vi "GeoData.vi"() -> ()   [LabVIEW 2017] (continued)
VA\tAppomattox County\tH1\n22205\t51013\tArlington\tVA\tArlington County\tH1\n22230\t51013\tArlington\tVA\tArlington County\tH1\n22203\t51013\tArlington\tVA\tArlington County\tH1\n22211\t51013\tFort myer\tVA\tArlington County\tH1\n20350\t51013\tWashington\tVA\tArlington County\tH1\n22217\t51013\tArlington\tVA\tArlington County\tH1\n20310\t51013\tWashington\tVA\tArlington County\tH1\n22225\t51013\tArlington\tVA\tArlington County\tH1\n22212\t51013\tArlington\tVA\tArlington County\tH1\n22101\t51013\tMc lean\tVA\tArlington County\tH1\n22202\t51013\tArlington\tVA\tArlington County\tH1\n22204\t51013\tArlington\tVA\tArlington County\tH1\n22243\t51013\tArlington\tVA\tArlington County\tH1\n22046\t51013\tFalls church\tVA\tArlington County\tH1\n22201\t51013\tArlington\tVA\tArlington County\tH1\n22240\t51013\tArlington\tVA\tArlington County\tH1\n20598\t51013\tDhs\tVA\tArlington County\tH1\n22213\t51013\tArlington\tVA\tArlington County\tH1\n22219\t51013\tArlington\tVA\tArlington County\tH1\n22214\t51013\tArlington\tVA\tArlington County\tH1\n22226\t51013\tArlington\tVA\tArlington County\tH1\n22206\t51013\tArlington\tVA\tArlington County\tH1\n22207\t51013\tArlington\tVA\tArlington County\tH1\n22216\t51013\tArlington\tVA\tArlington County\tH1\n22210\t51013\tArlington\tVA\tArlington County\tH1\n22242\t51013\tArlington\tVA\tArlington County\tH1\n22244\t51013\tArlington\tVA\tArlington County\tH1\n20406\t51013\tWashington\tVA\tArlington County\tH1\n22209\t51013\tArlington\tVA\tArlington County\tH1\n20330\t51013\tWashington\tVA\tArlington County\tH1\n22215\t51013\tArlington\tVA\tArlington County\tH1\n20301\t51013\tWashington\tVA\tArlington County\tH1\n22227\t51013\tArlington\tVA\tArlington County\tH1\n22245\t51013\tArlington\tVA\tArlington County\tH1\n22241\t51013\tArlington\tVA\tArlington County\tH1\n22920\t51015\tAfton\tVA\tAugusta County\tH1\n22967\t51015\tRoseland\tVA\tAugusta County\tH1\n24477\t51015\tStuarts draft\tVA\tAugusta County\tH1\n24437\t51015\tFort defiance\tVA\tAugusta County\tH1\n22843\t51015\tMount solon\tVA\tAugusta County\tH1\n22841\t51015\tMount crawford\tVA\tAugusta County\tH1\n24467\t51015\tMount sidney\tVA\tAugusta County\tH1\n24486\t51015\tWeyers cave\tVA\tAugusta County\tH1\n24482\t51015\tVerona\tVA\tAugusta County\tH1\n24483\t51015\tVesuvius\tVA\tAugusta County\tH1\n24440\t51015\tGreenville\tVA\tAugusta County\tH1\n24463\t51015\tMint spring\tVA\tAugusta County\tH1\n22812\t51015\tBridgewater\tVA\tAugusta County\tH1\n22980\t51015\tWaynesboro\tVA\tAugusta County\tH1\n24441\t51015\tGrottoes\tVA\tAugusta County\tH1\n24479\t51015\tSwoope\tVA\tAugusta County\tH1\n22952\t51015\tLyndhurst\tVA\tAugusta County\tH1\n24472\t51015\tRaphine\tVA\tAugusta County\tH1\n24411\t51015\tAugusta springs\tVA\tAugusta County\tH1\n24401\t51015\tStaunton\tVA\tAugusta County\tH1\n24459\t51015\tMiddlebrook\tVA\tAugusta County\tH1\n24421\t51015\tChurchville\tVA\tAugusta County\tH1\n22939\t51015\tFishersville\tVA\tAugusta County\tH1\n24485\t51015\tWest augusta\tVA\tAugusta County\tH1\n24430\t51015\tCraigsville\tVA\tAugusta County\tH1\n24476\t51015\tSteeles tavern\tVA\tAugusta County\tH1\n24469\t51015\tNew hope\tVA\tAugusta County\tH1\n24439\t51015\tGoshen\tVA\tAugusta County\tH1\n24432\t51015\tDeerfield\tVA\tAugusta County\tH1\n24431\t51015\tCrimora\tVA\tAugusta County\tH1\n24460\t51017\tMillboro\tVA\tBath County\tH1\n24422\t51017\tClifton forge\tVA\tBath County\tH1\n24445\t51017\tHot springs\tVA\tBath County\tH1\n24412\t51017\tBacova\tVA\tBath County\tH1\n24487\t51017\tWilliamsville\tVA\tBath County\tH1\n24484\t51017\tWarm springs\tVA\tBath County\tH1\n24432\t51017\tDeerfield\tVA\tBath County\tH1\n24104\t51019\tHuddleston\tVA\tBedford County\tH1\n24122\t51019\tMontvale\tVA\tBedford County\tH1\n24139\t51019\tPittsville\tVA\tBedford County\tH1\n24503\t51019\tLynchburg\tVA\tBedford County\tH1\n24536\t51019\tColeman falls\tVA\tBedford County\tH1\n24523\t51019\tBedford\tVA\tBedford County\tH1\n24550\t51019\tEvington\tVA\tBedford County\tH1\n24101\t51019\tHardy\tVA\tBedford County\tH1\n24179\t51019\tVinton\tVA\tBedford County\tH1\n24502\t51019\tLynchburg\tVA\tBedford County\tH1\n24570\t51019\tLowry\tVA\tBedford County\tH1\n24064\t51019\tBlue ridge\tVA\tBedford County\tH1\n24174\t51019\tThaxton\tVA\tBedford County\tH1\n24501\t51019\tLynchburg\tVA\tBedford County\tH1\n24556\t51019\tGoode\tVA\tBedford County\tH1\n24095\t51019\tGoodview\tVA\tBedford County\tH1\n24551\t51019\tForest\tVA\tBedford County\tH1\n24571\t51019\tLynch station\tVA\tBedford County\tH1\n24121\t51019\tMoneta\tVA\tBedford County\tH1\n24526\t51019\tBig island\tVA\tBedford County\tH1\n24084\t51021\tDublin\tVA\tBland County\tH1\n24315\t51021\tBland\tVA\tBland County\tH1\n24314\t51021\tBastian\tVA\tBland County\tH1\n24124\t51021\tNarrows\tVA\tBland County\tH1\n24134\t51021\tPearisburg\tVA\tBland County\tH1\n24366\t51021\tRocky gap\tVA\tBland County\tH1\n24318\t51021\tCeres\tVA\tBland County\tH1\n24012\t51023\tRoanoke\tVA\tBotetourt County\tH1\n24090\t51023\tFincastle\tVA\tBotetourt County\tH1\n24175\t51023\tTroutville\tVA\tBotetourt County\tH1\n24579\t51023\tNatural bridge station\tVA\tBotetourt County\tH1\n24066\t51023\tBuchanan\tVA\tBotetourt County\tH1\n24450\t51023\tLexington\tVA\tBotetourt County\tH1\n24085\t51023\tEagle rock\tVA\tBotetourt County\tH1\n24422\t51023\tClifton forge\tVA\tBotetourt County\tH1\n24077\t51023\tCloverdale\tVA\tBotetourt County\tH1\n24083\t51023\tDaleville\tVA\tBotetourt County\tH1\n24064\t51023\tBlue ridge\tVA\tBotetourt County\tH1\n24019\t51023\tRoanoke\tVA\tBotetourt County\tH1\n24155\t51023\tRoanoke\tVA\tBotetourt County\tH1\n24130\t51023\tOriskany\tVA\tBotetourt County\tH1\n24438\t51023\tGlen wilton\tVA\tBotetourt County\tH1\n23887\t51025\tValentines\tVA\tBrunswick County\tH1\n23843\t51025\tDolphin\tVA\tBrunswick County\tH1\n23845\t51025\tEbony\tVA\tBrunswick County\tH1\n23873\t51025\tMeredithville\tVA\tBrunswick County\tH1\n23919\t51025\tBracey\tVA\tBrunswick County\tH1\n23856\t51025\tFreeman\tVA\tBrunswick County\tH1\n23847\t51025\tEmporia\tVA\tBrunswick County\tH1\n23876\t51025\tRawlings\tVA\tBrunswick County\tH1\n23868\t51025\tLawrenceville\tVA\tBrunswick County\tH1\n23889\t51025\tWarfield\tVA\tBrunswick County\tH1\n23893\t51025\tWhite plains\tVA\tBrunswick County\tH1\n23920\t51025\tBrodnax\tVA\tBrunswick County\tH1\n23938\t51025\tDundas\tVA\tBrunswick County\tH1\n23824\t51025\tBlackstone\tVA\tBrunswick County\tH1\n23950\t51025\tLa crosse\tVA\tBrunswick County\tH1\n23857\t51025\tGasburg\tVA\tBrunswick County\tH1\n23821\t51025\tAlberta\tVA\tBrunswick County\tH1\n24634\t51027\tPilgrims knob\tVA\tBuchanan County\tH1\n24631\t51027\tOakwood\tVA\tBuchanan County\tH1\n24603\t51027\tBig rock\tVA\tBuchanan County\tH1\n24256\t51027\tHaysi\tVA\tBuchanan County\tH1\n24620\t51027\tHurley\tVA\tBuchanan County\tH1\n24622\t51027\tJewell ridge\tVA\tBuchanan County\tH1\n24656\t51027\tVansant\tVA\tBuchanan County\tH1\n24657\t51027\tWhitewood\tVA\tBuchanan County\tH1\n24639\t51027\tRaven\tVA\tBuchanan County\tH1\n24628\t51027\tMaxie\tVA\tBuchanan County\tH1\n24658\t51027\tWolford\tVA\tBuchanan County\tH1\n24614\t51027\tGrundy\tVA\tBuchanan County\tH1\n24260\t51027\tHonaker\tVA\tBuchanan County\tH1\n24217\t51027\tBee\tVA\tBuchanan County\tH1\n24649\t51027\tSwords creek\tVA\tBuchanan County\tH1\n24646\t51027\tRowe\tVA\tBuchanan County\tH1\n24239\t51027\tDavenport\tVA\tBuchanan County\tH1\n24624\t51027\tKeen mountain\tVA\tBuchanan County\tH1\n24627\t51027\tMavisdale\tVA\tBuchanan County\tH1\n23936\t51029\tDillwyn\tVA\tBuckingham County\tH1\n23921\t51029\tBuckingham\tVA\tBuckingham County\tH1\n24599\t51029\tWingina\tVA\tBuckingham County\tH1\n23901\t51029\tFarmville\tVA\tBuckingham County\tH1\n23004\t51029\tArvonia\tVA\tBuckingham County\tH1\n23123\t51029\tNew canton\tVA\tBuckingham County\tH1\n23040\t51029\tCumberland\tVA\tBuckingham County\tH1\n24522\t51029\tAppomattox\tVA\tBuckingham County\tH1\n24562\t51029\tHowardsville\tVA\tBuckingham County\tH1\n24553\t51029\tGladstone\tVA\tBuckingham County\tH1\n24590\t51029\tScottsville\tVA\tBuckingham County\tH1\n24504\t51031\tLynchburg\tVA\tCampbell County\tH1\n24588\t51031\tRustburg\tVA\tCampbell County\tH1\n24593\t51031\tSpout spring\tVA\tCampbell County\tH1\n24550\t51031\tEvington\tVA\tCampbell County\tH1\n24502\t51031\tLynchburg\tVA\tCampbell County\tH1\n24538\t51031\tConcord\tVA\tCampbell County\tH1\n24554\t51031\tGladys\tVA\tCampbell County\tH1\n24522\t51031\tAppomattox\tVA\tCampbell County\tH1\n24501\t51031\tLynchburg\tVA\tCampbell County\tH1\n24528\t51031\tBrookneal\tVA\tCampbell County\tH1\n24517\t51031\tAltavista\tVA\tCampbell County\tH1\n24576\t51031\tNaruna\tVA\tCampbell County\tH1\n24551\t51031\tForest\tVA\tCampbell County\tH1\n24569\t51031\tLong island\tVA\tCampbell County\tH1\n24571\t51031\tLynch station\tVA\tCampbell County\tH1\n23963\t51031\tRed house\tVA\tCampbell County\tH1\n22427\t51033\tBowling green\tVA\tCaroline County\tH1\n22438\t51033\tChamplain\tVA\tCaroline County\tH1\n22408\t51033\tFredericksburg\tVA\tCaroline County\tH1\n22514\t51033\tMilford\tVA\tCaroline County\tH1\n22560\t51033\tTappahannock\tVA\tCaroline County\tH1\n22436\t51033\tCaret\tVA\tCaroline County\tH1\n22535\t51033\tPort royal\tVA\tCaroline County\tH1\n22552\t51033\tSparta\tVA\tCaroline County\tH1\n22546\t51033\tRuther glen\tVA\tCaroline County\tH1\n22446\t51033\tCorbin\tVA\tCaroline County\tH1\n22580\t51033\tWoodford\tVA\tCaroline County\tH1\n22501\t51033\tLadysmith\tVA\tCaroline County\tH1\n23015\t51033\tBeaverdam\tVA\tCaroline County\tH1\n23047\t51033\tDoswell\tVA\tCaroline County\tH1\n22428\t51033\tBowling green\tVA\tCaroline County\tH1\n23069\t51033\tHanover\tVA\tCaroline County\tH1\n22538\t51033\tRappahannock academy\tVA\tCaroline County\tH1\n24330\t51035\tFries\tVA\tCarroll County\tH1\n24360\t51035\tMax meadows\tVA\tCarroll County\tH1\n24333\t51035\tGalax\tVA\tCarroll County\tH1\n24317\t51035\tCana\tVA\tCarroll County\tH1\n24328\t51035\tFancy gap\tVA\tCarroll County\tH1\n24352\t51035\tLaurel fork\tVA\tCarroll County\tH1\n24053\t51035\tArarat\tVA\tCarroll County\tH1\n24105\t51035\tIndian valley\tVA\tCarroll County\tH1\n24347\t51035\tHiwassee\tVA\tCarroll County\tH1\n24350\t51035\tIvanhoe\tVA\tCarroll County\tH1\n24343\t51035\tHillsville\tVA\tCarroll County\tH1\n24120\t51035\tMeadows of dan\tVA\tCarroll County\tH1\n24325\t51035\tDugspur\tVA\tCarroll County\tH1\n24312\t51035\tAustinville\tVA\tCarroll County\tH1\n24380\t51035\tWillis\tVA\tCarroll County\tH1\n24381\t51035\tWoodlawn\tVA\tCarroll County\tH1\n24351\t51035\tLambsburg\tVA\tCarroll County\tH1\n23030\t51036\tCharles city\tVA\tCharles City County\tH1\n23185\t51036\tWilliamsburg\tVA\tCharles City County\tH1\n23147\t51036\tRuthville\tVA\tCharles City County\tH1\n23231\t51036\tHenrico\tVA\tCharles City County\tH1\n23140\t51036\tProvidence forge\tVA\tCharles City County\tH1\n23937\t51037\tDrakes branch\tVA\tCharlotte County\tH1\n23959\t51037\tPhenix\tVA\tCharlotte County\tH1\n23967\t51037\tSaxe\tVA\tCharlotte County\tH1\n23962\t51037\tRandolph\tVA\tCharlotte County\tH1\n23947\t51037\tKeysville\tVA\tCharlotte County\tH1\n23934\t51037\tCullen\tVA\tCharlotte County\tH1\n23924\t51037\tChase city\tVA\tCharlotte County\tH1\n24522\t51037\tAppomattox\tVA\tCharlotte County\tH1\n24528\t51037\tBrookneal\tVA\tCharlotte County\tH1\n23964\t51037\tRed oak\tVA\tCharlotte County\tH1\n23927\t51037\tClarksville\tVA\tCharlotte County\tH1\n23976\t51037\tWylliesburg\tVA\tCharlotte County\tH1\n23923\t51037\tCharlotte court house\tVA\tCharlotte County\tH1\n23958\t51037\tPamplin\tVA\tCharlotte County\tH1\n23963\t51037\tRed house\tVA\tCharlotte County\tH1\n23224\t51041\tRichmond\tVA\tChesterfield County\tH1\n23235\t51041\tRichmond\tVA\tChesterfield County\tH1\n23834\t51041\tColonial heights\tVA\tChesterfield County\tH1\n23113\t51041\tMidlothian\tVA\tChesterfield County\tH1\n23114\t51041\tMidlothian\tVA\tChesterfield County\tH1\n23112\t51041\tMidlothian\tVA\tChesterfield County\tH1\n23236\t51041\tRichmond\tVA\tChesterfield County\tH1\n23803\t51041\tPetersburg\tVA\tChesterfield County\tH1\n23838\t51041\tChesterfield\tVA\tChesterfield County\tH1\n23120\t51041\tMoseley\tVA\tChesterfield County\tH1\n23832\t51041\tChesterfield\tVA\tChesterfield County\tH1\n23234\t51041\tRichmond\tVA\tChesterfield County\tH1\n23831\t51041\tChester\tVA\tChesterfield County\tH1\n23836\t51041\tChester\tVA\tChesterfield County\tH1\n23225\t51041\tRichmond\tVA\tChesterfield County\tH1\n23237\t51041\tRichmond\tVA\tChesterfield County\tH1\n23297\t51041\tRichmond\tVA\tChesterfield County\tH1\n22630\t51043\tFront royal\tVA\tClarke County\tH1\n20135\t51043\tBluemont\tVA\tClarke County\tH1\n20130\t51043\tParis\tVA\tClarke County\tH1\n22611\t51043\tBerryville\tVA\tClarke County\tH1\n22620\t51043\tBoyce\tVA\tClarke County\tH1\n22663\t51043\tWhite post\tVA\tClarke County\tH1\n22646\t51043\tMillwood\tVA\tClarke County\tH1\n24128\t51045\tNewport\tVA\tCraig County\tH1\n24127\t51045\tNew castle\tVA\tCraig County\tH1\n24070\t51045\tCatawba\tVA\tCraig County\tH1\n24131\t51045\tPaint bank\tVA\tCraig County\tH1\n24426\t51045\tCovington\tVA\tCraig County\tH1\n20186\t51047\tWarrenton\tVA\tCulpeper County\tH1\n22718\t51047\tElkwood\tVA\tCulpeper County\tH1\n22726\t51047\tLignum\tVA\tCulpeper County\tH1\n22714\t51047\tBrandy station\tVA\tCulpeper County\tH1\n20106\t51047\tAmissville\tVA\tCulpeper County\tH1\n22736\t51047\tRichardsville\tVA\tCulpeper County\tH1\n22733\t51047\tRapidan\tVA\tCulpeper County\tH1\n22729\t51047\tMitchells\tVA\tCulpeper County\tH1\n22716\t51047\tCastleton\tVA\tCulpeper County\tH1\n22724\t51047\tJeffersonton\tVA\tCulpeper County\tH1\n22713\t51047\tBoston\tVA\tCulpeper County\tH1\n22701\t51047\tCulpeper\tVA\tCulpeper County\tH1\n22735\t51047\tReva\tVA\tCulpeper County\tH1\n22734\t51047\tRemington\tVA\tCulpeper County\tH1\n22741\t51047\tStevensburg\tVA\tCulpeper County\tH1\n22740\t51047\tSperryville\tVA\tCulpeper County\tH1\n22407\t51047\tFredericksburg\tVA\tCulpeper County\tH1\n22737\t51047\tRixeyville\tVA\tCulpeper County\tH1\n23936\t51049\tDillwyn\tVA\tCumberland County\tH1\n23027\t51049\tCartersville\tVA\tCumberland County\tH1\n23901\t51049\tFarmville\tVA\tCumberland County\tH1\n23038\t51049\tColumbia\tVA\tCumberland County\tH1\n23123\t51049\tNew canton\tVA\tCumberland County\tH1\n23040\t51049\tCumberland\tVA\tCumberland County\tH1\n23139\t51049\tPowhatan\tVA\tCumberland County\tH1\n24237\t51051\tDante\tVA\tDickenson County\tH1\n24230\t51051\tCoeburn\tVA\tDickenson County\tH1\n24220\t51051\tBirchleaf\tVA\tDickenson County\tH1\n24226\t51051\tClinchco\tVA\tDickenson County\tH1\n24256\t51051\tHaysi\tVA\tDickenson County\tH1\n24225\t51051\tCleveland\tVA\tDickenson County\tH1\n24283\t51051\tSaint paul\tVA\tDickenson County\tH1\n24607\t51051\tBreaks\tVA\tDickenson County\tH1\n24656\t51051\tVansant\tVA\tDickenson County\tH1\n24228\t51051\tClintwood\tVA\tDickenson County\tH1\n24217\t51051\tBee\tVA\tDickenson County\tH1\n24272\t51051\tNora\tVA\tDickenson County\tH1\n24269\t51051\tMc clure\tVA\tDickenson County\tH1\n23833\t51053\tChurch road\tVA\tDinwiddie County\tH1\n23803\t51053\tPetersburg\tVA\tDinwiddie County\tH1\n23840\t51053\tDewitt\tVA\tDinwiddie County\tH1\n23805\t51053\tPetersburg\tVA\tDinwiddie County\tH1\n23885\t51053\tSutherland\tVA\tDinwiddie County\tH1\n23872\t51053\tMc kenney\tVA\tDinwiddie County\tH1\n23824\t51053\tBlackstone\tVA\tDinwiddie County\tH1\n23882\t51053\tStony creek\tVA\tDinwiddie County\tH1\n23894\t51053\tWilsons\tVA\tDinwiddie County\tH1\n23850\t51053\tFord\tVA\tDinwiddie County\tH1\n23830\t51053\tCarson\tVA\tDinwiddie County\tH1\n23841\t51053\tDinwiddie\tVA\tDinwiddie County\tH1\n22438\t51057\tChamplain\tVA\tEssex County\tH1\n23148\t51057\tSaint stephens church\tVA\tEssex County\tH1\n22454\t51057\tDunnsville\tVA\tEssex County\tH1\n22509\t51057\tLoretto\tVA\tEssex County\tH1\n22560\t51057\tTappahannock\tVA\tEssex County\tH1\n22436\t51057\tCaret\tVA\tEssex County\tH1\n23023\t51057\tBruington\tVA\tEssex County\tH1\n23115\t51057\tMillers tavern\tVA\tEssex County\tH1\n22437\t51057\tCenter cross\tVA\tEssex County\tH1\n22476\t51057\tHustle\tVA\tEssex County\tH1\n22504\t51057\tLaneview\tVA\tEssex County\tH1\n20171\t51059\tHerndon\tVA\tFairfax County\tH1\n22151\t51059\tSpringfield\tVA\tFairfax County\tH1\n22180\t51059\tVienna\tVA\tFairfax County\tH1\n22122\t51059\tNewington\tVA\tFairfax County\tH1\n22181\t51059\tVienna\tVA\tFairfax County\tH1\n22315\t51059\tAlexandria\tVA\tFairfax County\tH1\n22027\t51059\tDunn loring\tVA\tFairfax County\tH1\n22106\t51059\tMc lean\tVA\tFairfax County\tH1\n20195\t51059\tReston\tVA\tFairfax County\tH1\n22037\t51059\tFairfax\tVA\tFairfax County\tH1\n22158\t51059\tSpringfield\tVA\tFairfax County\tH1\n20192\t51059\tHerndon\tVA\tFairfax County\tH1\n20124\t51059\tClifton\tVA\tFairfax County\tH1\n20120\t51059\tCentreville\tVA\tFairfax County\tH1\n20164\t51059\tSterling\tVA\tFairfax County\tH1\n20191\t51059\tReston\tVA\tFairfax County\tH1\n22003\t51059\tAnnandale\tVA\tFairfax County\tH1\n22030\t51059\tFairfax\tVA\tFairfax County\tH1\n22043\t51059\tFalls church\tVA\tFairfax County\tH1\n22102\t51059\tMc lean\tVA\tFairfax County\tH1\n22308\t51059\tAlexandria\tVA\tFairfax County\tH1\n22121\t51059\tMount vernon\tVA\tFairfax County\tH1\n22035\t51059\tFairfax\tVA\tFairfax County\tH1\n22081\t51059\tMerrifield\tVA\tFairfax County\tH1\n22082\t51059\tMerrifield\tVA\tFairfax County\tH1\n22044\t51059\tFalls church\tVA\tFairfax County\tH1\n22183\t51059\tVienna\tVA\tFairfax County\tH1\n22312\t51059\tAlexandria\tVA\tFairfax County\tH1\n22159\t51059\tSpringfield\tVA\tFairfax County\tH1\n22108\t51059\tMc lean\tVA\tFairfax County\tH1\n20041\t51059\tWashington\tVA\tFairfax County\tH1\n22161\t51059\tSpringfield\tVA\tFairfax County\tH1\n20190\t51059\tReston\tVA\tFairfax County\tH1\n20194\t51059\tReston\tVA\tFairfax County\tH1\n22041\t51059\tFalls church\tVA\tFairfax County\tH1\n22101\t51059\tMc lean\tVA\tFairfax County\tH1\n22124\t51059\tOakton\tVA\tFairfax County\tH1\n22150\t51059\tSpringfield\tVA\tFairfax County\tH1\n22204\t51059\tArlington\tVA\tFairfax County\tH1\n22302\t51059\tAlexandria\tVA\tFairfax County\tH1\n22304\t51059\tAlexandria\tVA\tFairfax County\tH1\n22067\t51059\tGreenway\tVA\tFairfax County\tH1\n20152\t51059\tChantilly\tVA\tFairfax County\tH1\n20170\t51059\tHerndon\tVA\tFairfax County\tH1\n20165\t51059\tSterling\tVA\tFairfax County\tH1\n22046\t51059\tFalls church\tVA\tFairfax County\tH1\n22066\t51059\tGreat falls\tVA\tFairfax County\tH1\n22152\t51059\tSpringfield\tVA\tFairfax County\tH1\n22079\t51059\tLorton\tVA\tFairfax County\tH1\n22116\t51059\tMerrifield\tVA\tFairfax County\tH1\n22160\t51059\tSpringfield\tVA\tFairfax County\tH1\n20070\t51059\tWashington\tVA\tFairfax County\tH1\n20206\t51059\tWashington\tVA\tFairfax County\tH1\n20598\t51059\tDhs\tVA\tFairfax County\tH1\n20122\t51059\tCentreville\tVA\tFairfax County\tH1\n22009\t51059\tBurke\tVA\tFairfax County\tH1\n22039\t51059\tFairfax station\tVA\tFairfax County\tH1\n22303\t51059\tAlexandria\tVA\tFairfax County\tH1\n22306\t51059\tAlexandria\tVA\tFairfax County\tH1\n22213\t51059\tArlington\tVA\tFairfax County\tH1\n22103\t51059\tWest mclean\tVA\tFairfax County\tH1\n22185\t51059\tVienna\tVA\tFairfax County\tH1\n20121\t51059\tCentreville\tVA\tFairfax County\tH1\n20153\t51059\tChantilly\tVA\tFairfax County\tH1\n22015\t51059\tBurke\tVA\tFairfax County\tH1\n22031\t51059\tFairfax\tVA\tFairfax County\tH1\n22042\t51059\tFalls church\tVA\tFairfax County\tH1\n22153\t51059\tSpringfield\tVA\tFairfax County\tH1\n22060\t51059\tFort belvoir\tVA\tFairfax County\tH1\n22206\t51059\tArlington\tVA\tFairfax County\tH1\n22207\t51059\tArlington\tVA\tFairfax County\tH1\n22310\t51059\tAlexandria\tVA\tFairfax County\tH1\n22199\t51059\tLorton\tVA\tFairfax County\tH1\n22107\t51059\tMc lean\tVA\tFairfax County\tH1\n20151\t51059\tChantilly\tVA\tFairfax County\tH1\n22033\t51059\tFairfax\tVA\tFairfax County\tH1\n22032\t51059\tFairfax\tVA\tFairfax County\tH1\n22182\t51059\tVienna\tVA\tFairfax County\tH1\n22307\t51059\tAlexandria\tVA\tFairfax County\tH1\n22311\t51059\tAlexandria\tVA\tFairfax County\tH1\n22309\t51059\tAlexandria\tVA\tFairfax County\tH1\n20172\t51059\tHerndon\tVA\tFairfax County\tH1\n22109\t51059\tMc lean\tVA\tFairfax County\tH1\n20069\t51059\tWashington\tVA\tFairfax County\tH1\n22406\t51061\tFredericksburg\tVA\tFauquier County\tH1\n20128\t51061\tOrlean\tVA\tFauquier County\tH1\n20139\t51061\tCasanova\tVA\tFauquier County\tH1\n20115\t51061\tMarshall\tVA\tFauquier County\tH1\n20186\t51061\tWarrenton\tVA\tFauquier County\tH1\n20181\t51061\tNokesville\tVA\tFauquier County\tH1\n22639\t51061\tHume\tVA\tFauquier County\tH1\n20106\t51061\tAmissville\tVA\tFauquier County\tH1\n22720\t51061\tGoldvein\tVA\tFauquier County\tH1\n22556\t51061\tStafford\tVA\tFauquier County\tH1\n20144\t51061\tDelaplane\tVA\tFauquier County\tH1\n20137\t51061\tBroad run\tVA\tFauquier County\tH1\n22642\t51061\tLinden\tVA\tFauquier County\tH1\n20138\t51061\tCalverton\tVA\tFauquier County\tH1\n20130\t51061\tParis\tVA\tFauquier County\tH1\n20169\t51061\tHaymarket\tVA\tFauquier County\tH1\n22643\t51061\tMarkham\tVA\tFauquier County\tH1\n22712\t51061\tBealeton\tVA\tFauquier County\tH1\n22734\t51061\tRemington\tVA\tFauquier County\tH1\n22728\t51061\tMidland\tVA\tFauquier County\tH1\n20198\t51061\tThe plains\tVA\tFauquier County\tH1\n20184\t51061\tUpperville\tVA\tFauquier County\tH1\n20188\t51061\tWarrenton\tVA\tFauquier County\tH1\n20140\t51061\tRectortown\tVA\tFauquier County\tH1\n20117\t51061\tMiddleburg\tVA\tFauquier County\tH1\n20187\t51061\tWarrenton\tVA\tFauquier County\tH1\n22742\t51061\tSumerduck\tVA\tFauquier County\tH1\n20119\t51061\tCatlett\tVA\tFauquier County\tH1\n24091\t51063\tFloyd\tVA\tFloyd County\tH1\n24149\t51063\tRiner\tVA\tFloyd County\tH1\n24352\t51063\tLaurel fork\tVA\tFloyd County\tH1\n24059\t51063\tBent mountain\tVA\tFloyd County\tH1\n24079\t51063\tCopper hill\tVA\tFloyd County\tH1\n24105\t51063\tIndian valley\tVA\tFloyd County\tH1\n24141\t51063\tRadford\tVA\tFloyd County\tH1\n24162\t51063\tShawsville\tVA\tFloyd County\tH1\n24120\t51063\tMeadows of dan\tVA\tFloyd County\tH1\n24138\t51063\tPilot\tVA\tFloyd County\tH1\n24380\t51063\tWillis\tVA\tFloyd County\tH1\n24072\t51063\tCheck\tVA\tFloyd County\tH1\n22963\t51065\tPalmyra\tVA\tFluvanna County\tH1\n23055\t51065\tFork union\tVA\tFluvanna County\tH1\n23093\t51065\tLouisa\tVA\tFluvanna County\tH1\n22947\t51065\tKeswick\tVA\tFluvanna County\tH1\n23038\t51065\tColumbia\tVA\tFluvanna County\tH1\n23084\t51065\tKents store\tVA\tFluvanna County\tH1\n22974\t51065\tTroy\tVA\tFluvanna County\tH1\n23022\t51065\tBremo bluff\tVA\tFluvanna County\tH1\n24590\t51065\tScottsville\tVA\tFluvanna County\tH1\n24014\t51067\tRoanoke\tVA\tFranklin County\tH1\n24146\t51067\tRedwood\tVA\tFranklin County\tH1\n24055\t51067\tBassett\tVA\tFranklin County\tH1\n24065\t51067\tBoones mill\tVA\tFranklin County\tH1\n24091\t51067\tFloyd\tVA\tFranklin County\tH1\n24092\t51067\tGlade hill\tVA\tFranklin County\tH1\n24112\t51067\tMartinsville\tVA\tFranklin County\tH1\n24059\t51067\tBent mountain\tVA\tFranklin County\tH1\n24079\t51067\tCopper hill\tVA\tFranklin County\tH1\n24088\t51067\tFerrum\tVA\tFranklin County\tH1\n24101\t51067\tHardy\tVA\tFranklin County\tH1\n24102\t51067\tHenry\tVA\tFranklin County\tH1\n24151\t51067\tRocky mount\tVA\tFranklin County\tH1\n24067\t51067\tCallaway\tVA\tFranklin County\tH1\n24137\t51067\tPenhook\tVA\tFranklin County\tH1\n24184\t51067\tWirtz\tVA\tFranklin County\tH1\n24121\t51067\tMoneta\tVA\tFranklin County\tH1\n24176\t51067\tUnion hall\tVA\tFranklin County\tH1\n22601\t51069\tWinchester\tVA\tFrederick County\tH1\n22630\t51069\tFront royal\tVA\tFrederick County\tH1\n22645\t51069\tMiddletown\tVA\tFrederick County\tH1\n22624\t51069\tClear brook\tVA\tFrederick County\tH1\n22602\t51069\tWinchester\tVA\tFrederick County\tH1\n22622\t51069\tBrucetown\tVA\tFrederick County\tH1\n22637\t51069\tGore\tVA\tFrederick County\tH1\n22656\t51069\tStephenson\tVA\tFrederick County\tH1\n22655\t51069\tStephens city\tVA\tFrederick County\tH1\n22654\t51069\tStar tannery\tVA\tFrederick County\tH1\n22625\t51069\tCross junction\tVA\tFrederick County\tH1\n22603\t51069\tWinchester\tVA\tFrederick County\tH1\n22663\t51069\tWhite post\tVA\tFrederick County\tH1\n24315\t51071\tBland\tVA\tGiles County\tH1\n24147\t51071\tRich creek\tVA\tGiles County\tH1\n24128\t51071\tNewport\tVA\tGiles County\tH1\n24150\t51071\tRipplemead\tVA\tGiles County\tH1\n24136\t51071\tPembroke\tVA\tGiles County\tH1\n24124\t51071\tNarrows\tVA\tGiles County\tH1\n24134\t51071\tPearisburg\tVA\tGiles County\tH1\n24086\t51071\tEggleston\tVA\tGiles County\tH1\n24167\t51071\tStaffordsville\tVA\tGiles County\tH1\n24093\t51071\tGlen lyn\tVA\tGiles County\tH1\n23001\t51073\tAchilles\tVA\tGloucester County\tH1\n23154\t51073\tSchley\tVA\tGloucester County\tH1\n23155\t51073\tSevern\tVA\tGloucester County\tH1\n23072\t51073\tHayes\tVA\tGloucester County\tH1\n23183\t51073\tWhite marsh\tVA\tGloucester County\tH1\n23003\t51073\tArk\tVA\tGloucester County\tH1\n23018\t51073\tBena\tVA\tGloucester County\tH1\n23128\t51073\tNorth\tVA\tGloucester County\tH1\n23131\t51073\tOrdinary\tVA\tGloucester County\tH1\n23184\t51073\tWicomico\tVA\tGloucester County\tH1\n23061\t51073\tGloucester\tVA\tGloucester County\tH1\n23050\t51073\tDutton\tVA\tGloucester County\tH1\n23062\t51073\tGloucester point\tVA\tGloucester County\tH1\n23149\t51073\tSaluda\tVA\tGloucester County\tH1\n23190\t51073\tWoods cross roads\tVA\tGloucester County\tH1\n23178\t51073\tWare neck\tVA\tGloucester County\tH1\n23065\t51075\tGum spring\tVA\tGoochland County\tH1\n23093\t51075\tLouisa\tVA\tGoochland County\tH1\n23059\t51075\tGlen allen\tVA\tGoochland County\tH1\n23117\t51075\tMineral\tVA\tGoochland County\tH1\n23102\t51075\tMaidens\tVA\tGoochland County\tH1\n23067\t51075\tHadensville\tVA\tGoochland County\tH1\n23233\t51075\tHenrico\tVA\tGoochland County\tH1\n23039\t51075\tCrozier\tVA\tGoochland County\tH1\n23129\t51075\tOilville\tVA\tGoochland County\tH1\n23160\t51075\tState farm\tVA\tGoochland County\tH1\n23063\t51075\tGoochland\tVA\tGoochland County\tH1\n23038\t51075\tColumbia\tVA\tGoochland County\tH1\n23103\t51075\tManakin sabot\tVA\tGoochland County\tH1\n23153\t51075\tSandy hook\tVA\tGoochland County\tH1\n23146\t51075\tRockville\tVA\tGoochland County\tH1\n23238\t51075\tHenrico\tVA\tGoochland County\tH1\n23084\t51075\tKents store\tVA\tGoochland County\tH1\n24330\t51077\tFries\tVA\tGrayson County\tH1\n24333\t51077\tGalax\tVA\tGrayson County\tH1\n24326\t51077\tElk creek\tVA\tGrayson County\tH1\n24348\t51077\tIndependence\tVA\tGrayson County\tH1\n24363\t51077\tMouth of wilson\tVA\tGrayson County\tH1\n24350\t51077\tIvanhoe\tVA\tGrayson County\tH1\n24430\t51077\tCraigsville\tVA\tGrayson County\tH1\n24292\t51077\tWhitetop\tVA\tGrayson County\tH1\n24378\t51077\tTroutdale\tVA\tGrayson County\tH1\n22935\t51079\tDyke\tVA\tGreene County\tH1\n22940\t51079\tFree union\tVA\tGreene County\tH1\n22965\t51079\tQuinque\tVA\tGreene County\tH1\n22923\t51079\tBarboursville\tVA\tGreene County\tH1\n22936\t51079\tEarlysville\tVA\tGreene County\tH1\n22968\t51079\tRuckersville\tVA\tGreene County\tH1\n22973\t51079\tStanardsville\tVA\tGreene County\tH1\n23887\t51081\tValentines\tVA\tGreensville County\tH1\n23867\t51081\tJarratt\tVA\tGreensville County\tH1\n23856\t51081\tFreeman\tVA\tGreensville County\tH1\n23847\t51081\tEmporia\tVA\tGreensville County\tH1\n23870\t51081\tJarratt\tVA\tGreensville County\tH1\n23879\t51081\tSkippers\tVA\tGreensville County\tH1\n24534\t51083\tClover\tVA\tHalifax County\tH1\n24565\t51083\tJava\tVA\tHalifax County\tH1\n24594\t51083\tSutherlin\tVA\tHalifax County\tH1\n24577\t51083\tNathalie\tVA\tHalifax County\tH1\n24558\t51083\tHalifax\tVA\tHalifax County\tH1\n24520\t51083\tAlton\tVA\tHalifax County\tH1\n24539\t51083\tCrystal hill\tVA\tHalifax County\tH1\n23962\t51083\tRandolph\tVA\tHalifax County\tH1\n24597\t51083\tVernon hill\tVA\tHalifax County\tH1\n24598\t51083\tVirgilina\tVA\tHalifax County\tH1\n24529\t51083\tBuffalo junction\tVA\tHalifax County\tH1\n24589\t51083\tScottsburg\tVA\tHalifax County\tH1\n24557\t51083\tGretna\tVA\tHalifax County\tH1\n24569\t51083\tLong island\tVA\tHalifax County\tH1\n24592\t51083\tSouth boston\tVA\tHalifax County\tH1\n24535\t51083\tCluster springs\tVA\tHalifax County\tH1\n23059\t51085\tGlen allen\tVA\tHanover County\tH1\n23116\t51085\tMechanicsville\tVA\tHanover County\tH1\n23102\t51085\tMaidens\tVA\tHanover County\tH1\n23192\t51085\tMontpelier\tVA\tHanover County\tH1\n23129\t51085\tOilville\tVA\tHanover County\tH1\n23162\t51085\tStudley\tVA\tHanover County\tH1\n22546\t51085\tRuther glen\tVA\tHanover County\tH1\n23005\t51085\tAshland\tVA\tHanover County\tH1\n23124\t51085\tNew kent\tVA\tHanover County\tH1\n23015\t51085\tBeaverdam\tVA\tHanover County\tH1\n23047\t51085\tDoswell\tVA\tHanover County\tH1\n23111\t51085\tMechanicsville\tVA\tHanover County\tH1\n23146\t51085\tRockville\tVA\tHanover County\tH1\n23024\t51085\tBumpass\tVA\tHanover County\tH1\n23069\t51085\tHanover\tVA\tHanover County\tH1\n23030\t51087\tCharles city\tVA\tHenrico County\tH1\n23222\t51087\tRichmond\tVA\tHenrico County\tH1\n23229\t51087\tHenrico\tVA\tHenrico County\tH1\n23059\t51087\tGlen allen\tVA\tHenrico County\tH1\n23060\t51087\tGlen allen\tVA\tHenrico County\tH1\n23231\t51087\tHenrico\tVA\tHenrico County\tH1\n23294\t51087\tHenrico\tVA\tHenrico County\tH1\n23058\t51087\tGlen allen\tVA\tHenrico County\tH1\n23250\t51087\tRichmond\tVA\tHenrico County\tH1\n23150\t51087\tSandston\tVA\tHenrico County\tH1\n23233\t51087\tHenrico\tVA\tHenrico County\tH1\n23255\t51087\tHenrico\tVA\tHenrico County\tH1\n23227\t51087\tRichmond\tVA\tHenrico County\tH1\n23242\t51087\tHenrico\tVA\tHenrico County\tH1\n23223\t51087\tRichmond\tVA\tHenrico County\tH1\n23273\t51087\tHenrico\tVA\tHenrico County\tH1\n23075\t51087\tHenrico\tVA\tHenrico County\tH1\n23226\t51087\tRichmond\tVA\tHenrico County\tH1\n23228\t51087\tHenrico\tVA\tHenrico County\tH1\n23230\t51087\tRichmond\tVA\tHenrico County\tH1\n23238\t51087\tHenrico\tVA\tHenrico County\tH1\n24133\t51089\tPatrick springs\tVA\tHenry County\tH1\n24055\t51089\tBassett\tVA\tHenry County\tH1\n24078\t51089\tCollinsville\tVA\tHenry County\tH1\n24112\t51089\tMartinsville\tVA\tHenry County\tH1\n24054\t51089\tAxton\tVA\tHenry County\tH1\n24165\t51089\tSpencer\tVA\tHenry County\tH1\n24168\t51089\tStanleytown\tVA\tHenry County\tH1\n24102\t51089\tHenry\tVA\tHenry County\tH1\n24148\t51089\tRidgeway\tVA\tHenry County\tH1\n24530\t51089\tCallands\tVA\tHenry County\tH1\n24089\t51089\tFieldale\tVA\tHenry County\tH1\n24413\t51091\tBlue grass\tVA\tHighland County\tH1\n24442\t51091\tHead waters\tVA\tHighland County\tH1\n24465\t51091\tMonterey\tVA\tHighland County\tH1\n24433\t51091\tDoe hill\tVA\tHighland County\tH1\n24487\t51091\tWilliamsville\tVA\tHighland County\tH1\n24468\t51091\tMustoe\tVA\tHighland County\tH1\n24458\t51091\tMc dowell\tVA\tHighland County\tH1\n24484\t51091\tWarm springs\tVA\tHighland County\tH1\n23314\t51093\tCarrollton\tVA\tIsle of Wight County\tH1\n23432\t51093\tSuffolk\tVA\tIsle of Wight County\tH1\n23424\t51093\tRescue\tVA\tIsle of Wight County\tH1\n23397\t51093\tIsle of wight\tVA\tIsle of Wight County\tH1\n23487\t51093\tWindsor\tVA\tIsle of Wight County\tH1\n23851\t51093\tFranklin\tVA\tIsle of Wight County\tH1\n23898\t51093\tZuni\tVA\tIsle of Wight County\tH1\n23304\t51093\tBattery park\tVA\tIsle of Wight County\tH1\n23315\t51093\tCarrsville\tVA\tIsle of Wight County\tH1\n23430\t51093\tSmithfield\tVA\tIsle of Wight County\tH1\n23431\t51093\tSmithfield\tVA\tIsle of Wight County\tH1\n23866\t51093\tIvor\tVA\tIsle of Wight County\tH1\n23185\t51095\tWilliamsburg\tVA\tJames City County\tH1\n23081\t51095\tJamestown\tVA\tJames City County\tH1\n23188\t51095\tWilliamsburg\tVA\tJames City County\tH1\n23089\t51095\tLanexa\tVA\tJames City County\tH1\n23168\t51095\tToano\tVA\tJames City County\tH1\n23127\t51095\tNorge\tVA\tJames City County\tH1\n23156\t51097\tShacklefords\tVA\tKing and Queen County\tH1\n23148\t51097\tSaint stephens church\tVA\tKing and Queen County\tH1\n22514\t51097\tMilford\tVA\tKing and Queen County\tH1\n22560\t51097\tTappahannock\tVA\tKing and Queen County\tH1\n23023\t51097\tBruington\tVA\tKing and Queen County\tH1\n23126\t51097\tNewtown\tVA\tKing and Queen County\tH1\n22437\t51097\tCenter cross\tVA\tKing and Queen County\tH1\n23091\t51097\tLittle plymouth\tVA\tKing and Queen County\tH1\n23181\t51097\tWest point\tVA\tKing and Queen County\tH1\n23108\t51097\tMascot\tVA\tKing and Queen County\tH1\n23177\t51097\tWalkerton\tVA\tKing and Queen County\tH1\n23110\t51097\tMattaponi\tVA\tKing and Queen County\tH1\n23149\t51097\tSaluda\tVA\tKing and Queen County\tH1\n23085\t51097\tKing and queen court house\tVA\tKing and Queen County\tH1\n23161\t51097\tStevensville\tVA\tKing and Queen County\tH1\n22451\t51099\tDogue\tVA\tKing George County\tH1\n22448\t51099\tDahlgren\tVA\tKing George County\tH1\n22443\t51099\tColonial beach\tVA\tKing George County\tH1\n22485\t51099\tKing george\tVA\tKing George County\tH1\n22544\t51099\tRollins fork\tVA\tKing George County\tH1\n22481\t51099\tJersey\tVA\tKing George County\tH1\n22547\t51099\tSealston\tVA\tKing George County\tH1\n22526\t51099\tNinde\tVA\tKing George County\tH1\n23086\t51101\tKing william\tVA\tKing William County\tH1\n23009\t51101\tAylett\tVA\tKing William County\tH1\n23181\t51101\tWest point\tVA\tKing William County\tH1\n23106\t51101\tManquin\tVA\tKing William County\tH1\n23069\t51101\tHanover\tVA\tKing William County\tH1\n23177\t51101\tWalkerton\tVA\tKing William County\tH1\n22523\t51103\tMorattico\tVA\tLancaster County\tH1\n22578\t51103\tWhite stone\tVA\tLancaster County\tH1\n22576\t51103\tWeems\tVA\tLancaster County\tH1\n22482\t51103\tKilmarnock\tVA\tLancaster County\tH1\n22503\t51103\tLancaster\tVA\tLancaster County\tH1\n22480\t51103\tIrvington\tVA\tLancaster County\tH1\n22528\t51103\tNuttsville\tVA\tLancaster County\tH1\n22473\t51103\tHeathsville\tVA\tLancaster County\tH1\n22517\t51103\tMollusk\tVA\tLancaster County\tH1\n22513\t51103\tMerry point\tVA\tLancaster County\tH1\n22507\t51103\tLively\tVA\tLancaster County\tH1\n24219\t51105\tBig stone gap\tVA\tLee County\tH1\n24221\t51105\tBlackwater\tVA\tLee County\tH1\n24243\t51105\tDryden\tVA\tLee County\tH1\n24248\t51105\tEwing\tVA\tLee County\tH1\n24265\t51105\tKeokee\tVA\tLee County\tH1\n24281\t51105\tRose hill\tVA\tLee County\tH1\n24277\t51105\tPennington gap\tVA\tLee County\tH1\n24282\t51105\tSaint charles\tVA\tLee County\tH1\n24218\t51105\tBen hur\tVA\tLee County\tH1\n24263\t51105\tJonesville\tVA\tLee County\tH1\n24244\t51105\tDuffield\tVA\tLee County\tH1\n20160\t51107\tLincoln\tVA\tLoudoun County\tH1\n20135\t51107\tBluemont\tVA\tLoudoun County\tH1\n20141\t51107\tRound hill\tVA\tLoudoun County\tH1\n20120\t51107\tCentreville\tVA\tLoudoun County\tH1\n20164\t51107\tSterling\tVA\tLoudoun County\tH1\n20166\t51107\tSterling\tVA\tLoudoun County\tH1\n20129\t51107\tPaeonian springs\tVA\tLoudoun County\tH1\n20101\t51107\tDulles\tVA\tLoudoun County\tH1\n20132\t51107\tPurcellville\tVA\tLoudoun County\tH1\n20167\t51107\tSterling\tVA\tLoudoun County\tH1\n20149\t51107\tAshburn\tVA\tLoudoun County\tH1\n20189\t51107\tDulles\tVA\tLoudoun County\tH1\n20175\t51107\tLeesburg\tVA\tLoudoun County\tH1\n20159\t51107\tHamilton\tVA\tLoudoun County\tH1\n20152\t51107\tChantilly\tVA\tLoudoun County\tH1\n20147\t51107\tAshburn\tVA\tLoudoun County\tH1\n20165\t51107\tSterling\tVA\tLoudoun County\tH1\n20177\t51107\tLeesburg\tVA\tLoudoun County\tH1\n20178\t51107\tLeesburg\tVA\tLoudoun County\tH1\n22066\t51107\tGreat falls\tVA\tLoudoun County\tH1\n20158\t51107\tHamilton\tVA\tLoudoun County\tH1\n20598\t51107\tDhs\tVA\tLoudoun County\tH1\n20148\t51107\tAshburn\tVA\tLoudoun County\tH1\n20130\t51107\tParis\tVA\tLoudoun County\tH1\n20184\t51107\tUpperville\tVA\tLoudoun County\tH1\n20197\t51107\tWaterford\tVA\tLoudoun County\tH1\n20104\t51107\tDulles\tVA\tLoudoun County\tH1\n20103\t51107\tDulles\tVA\tLoudoun County\tH1\n20117\t51107\tMiddleburg\tVA\tLoudoun County\tH1\n20176\t51107\tLeesburg\tVA\tLoudoun County\tH1\n20146\t51107\tAshburn\tVA\tLoudoun County\tH1\n20105\t51107\tAldie\tVA\tLoudoun County\tH1\n20151\t51107\tChantilly\tVA\tLoudoun County\tH1\n20180\t51107\tLovettsville\tVA\tLoudoun County\tH1\n20131\t51107\tPhilomont\tVA\tLoudoun County\tH1\n23065\t51109\tGum spring\tVA\tLouisa County\tH1\n23093\t51109\tLouisa\tVA\tLouisa County\tH1\n23117\t51109\tMineral\tVA\tLouisa County\tH1\n23102\t51109\tMaidens\tVA\tLouisa County\tH1\n22942\t51109\tGordonsville\tVA\tLouisa County\tH1\n23192\t51109\tMontpelier\tVA\tLouisa County\tH1\n22947\t51109\tKeswick\tVA\tLouisa County\tH1\n23015\t51109\tBeaverdam\tVA\tLouisa County\tH1\n23084\t51109\tKents store\tVA\tLouisa County\tH1\n23170\t51109\tTrevilians\tVA\tLouisa County\tH1\n22974\t51109\tTroy\tVA\tLouisa County\tH1\n23024\t51109\tBumpass\tVA\tLouisa County\tH1\n23944\t51111\tKenbridge\tVA\tLunenburg County\tH1\n23952\t51111\tLunenburg\tVA\tLunenburg County\tH1\n23937\t51111\tDrakes branch\tVA\tLunenburg County\tH1\n23974\t51111\tVictoria\tVA\tLunenburg County\tH1\n23947\t51111\tKeysville\tVA\tLunenburg County\tH1\n23920\t51111\tBrodnax\tVA\tLunenburg County\tH1\n23970\t51111\tSouth hill\tVA\tLunenburg County\tH1\n23942\t51111\tGreen bay\tVA\tLunenburg County\tH1\n23938\t51111\tDundas\tVA\tLunenburg County\tH1\n23824\t51111\tBlackstone\tVA\tLunenburg County\tH1\n23924\t51111\tChase city\tVA\tLunenburg County\tH1\n23954\t51111\tMeherrin\tVA\tLunenburg County\tH1\n23923\t51111\tCharlotte court house\tVA\tLunenburg County\tH1\n22709\t51113\tAroda\tVA\tMadison County\tH1\n22732\t51113\tRadiant\tVA\tMadison County\tH1\n22948\t51113\tLocust dale\tVA\tMadison County\tH1\n22989\t51113\tWoodberry forest\tVA\tMadison County\tH1\n22715\t51113\tBrightwood\tVA\tMadison County\tH1\n22723\t51113\tHood\tVA\tMadison County\tH1\n22972\t51113\tSomerset\tVA\tMadison County\tH1\n22748\t51113\tWolftown\tVA\tMadison County\tH1\n22733\t51113\tRapidan\tVA\tMadison County\tH1\n22743\t51113\tSyria\tVA\tMadison County\tH1\n22722\t51113\tHaywood\tVA\tMadison County\tH1\n22701\t51113\tCulpeper\tVA\tMadison County\tH1\n22735\t51113\tReva\tVA\tMadison County\tH1\n22731\t51113\tPratts\tVA\tMadison County\tH1\n22719\t51113\tEtlan\tVA\tMadison County\tH1\n22740\t51113\tSperryville\tVA\tMadison County\tH1\n22725\t51113\tLeon\tVA\tMadison County\tH1\n22738\t51113\tRochelle\tVA\tMadison County\tH1\n22711\t51113\tBanco\tVA\tMadison County\tH1\n22727\t51113\tMadison\tVA\tMadison County\tH1\n22730\t51113\tOakpark\tVA\tMadison County\tH1\n22960\t51113\tOrange\tVA\tMadison County\tH1\n22973\t51113\tStanardsville\tVA\tMadison County\tH1\n23068\t51115\tHallieford\tVA\tMathews County\tH1\n23066\t51115\tGwynn\tVA\tMathews County\tH1\n23109\t51115\tMathews\tVA\tMathews County\tH1\n23130\t51115\tOnemo\tVA\tMathews County\tH1\n23035\t51115\tCobbs creek\tVA\tMathews County\tH1\n23125\t51115\tNew point\tVA\tMathews County\tH1\n23138\t51115\tPort haywood\tVA\tMathews County\tH1\n23045\t51115\tDiggs\tVA\tMathews County\tH1\n23025\t51115\tCardinal\tVA\tMathews County\tH1\n23076\t51115\tHudgins\tVA\tMathews County\tH1\n23128\t51115\tNorth\tVA\tMathews County\tH1\n23021\t51115\tBohannon\tVA\tMathews County\tH1\n23056\t51115\tFoster\tVA\tMathews County\tH1\n23050\t51115\tDutton\tVA\tMathews County\tH1\n23163\t51115\tSusan\tVA\tMathews County\tH1\n23119\t51115\tMoon\tVA\tMathews County\tH1\n23064\t51115\tGrimstead\tVA\tMathews County\tH1\n23919\t51117\tBracey\tVA\tMecklenburg County\tH1\n23968\t51117\tSkipwith\tVA\tMecklenburg County\tH1\n24598\t51117\tVirgilina\tVA\tMecklenburg County\tH1\n23920\t51117\tBrodnax\tVA\tMecklenburg County\tH1\n23970\t51117\tSouth hill\tVA\tMecklenburg County\tH1\n24580\t51117\tNelson\tVA\tMecklenburg County\tH1\n23917\t51117\tBoydton\tVA\tMecklenburg County\tH1\n23924\t51117\tChase city\tVA\tMecklenburg County\tH1\n24529\t51117\tBuffalo junction\tVA\tMecklenburg County\tH1\n23950\t51117\tLa crosse\tVA\tMecklenburg County\tH1\n23964\t51117\tRed oak\tVA\tMecklenburg County\tH1\n23927\t51117\tClarksville\tVA\tMecklenburg County\tH1\n23941\t51117\tFort mitchell\t
